vi "m1m3_ackCommand_Disable.vi"(8 "error in (no error)":errorcluster, 11 "ackcmd_Ctl":T1={"cmdSeqNum"=0, "ack"=0, "error"=0, "result"="                                                                                                                                                                                                                                                                "}) -> (0 "error out":errorcluster, 2 "function return":i32, 3 "ackcmd_Ctl out":T1={"cmdSeqNum"=0, "ack"=0, "error"=0, "result"="                                                                                                                                                                                                                                                                "})   [LabVIEW 2016, in "SALLV_m1m3.lvlib"]
doc: "int m1m3_shm_ackCommand_DisableLV(m1m3_ackcmdLV *ackcmd_Ctl);"
uses:
  SALLV_m1m3.lvlib
  DataTypes/ackcmd.ctl
  SALLV_m1m3.so
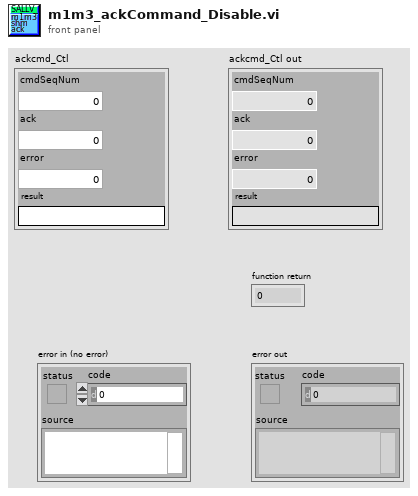
[diagram p1: front panel]
types:
  T1 = typedef "SALLV_m1m3.lvlib/ackcmd.ctl" = cluster{"cmdSeqNum":i32, "ack":i32, "error":i32, "result":string}
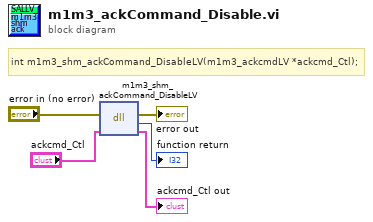
[diagram p0: block diagram]
diagram:
  # "int m1m3_shm_ackCommand_DisableLV(m1m3_ackcmdLV *ackcmd_Ctl);"
  n1 = dll-call lib="opt/CODE/ts_m1m3supporteui/SALLV_m1m3/SALLV_m1m3.*" fn="m1m3_shm_ackCommand_DisableLV"(error in="error in (no error)", "ackcmd_Ctl"="ackcmd_Ctl") -> (error out=→"error out":errorcluster, →"function return":i32, "ackcmd_Ctl"=→"ackcmd_Ctl out":T1)  [unwired: 2 in, 1 out]
